vi "string space.vi"() -> ()   [LabVIEW 2017]
uses:
  <vilib>/Utility/error.llb/whitespace.ctl
panel:
  out "length 2":i32
  out "length":i32
  out "trimmed string":string
  in  "String":string
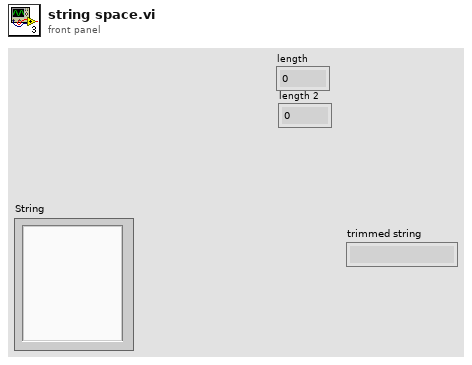
[diagram p1: front panel]
types:
  T1 = typedef "whitespace.ctl" = u16
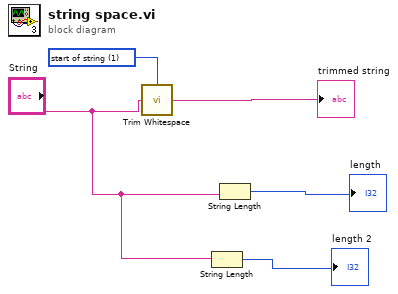
[diagram p0: block diagram]
diagram:
  w4 = T1 1 items=["both", "start of string", "end of string"] ("location (both)")
  n1 = call <vilib>:"Trim Whitespace.vi"("string"="String", "location (both)"=w4) -> ("trimmed string"=→"trimmed string":string)
  n2 = String Length(string="String") -> (length=→"length 2":i32)
  n3 = String Length(string="String") -> (length=→"length":i32)
